vi "Test PJVS.vi"(8 "error in (pass through)":errorcluster, 11 "PJVS setup":T1={"PJVS type"=enum."AC-supraVOLTcontrol", "Status Refnum"=refnum, "Abort Refnum"=refnum, "AC-supraVOLTcontrol"={"IP address:port (0.0.0.0:0000)"="0.0.0.0:0000", "Timeouts"={"TCP Read & Write (ms)"=7000, "Sensors readout"=5000, "PJVS setup"=10000, "Nullmeter readout"=5000, "Multiplexer setup"=3000, "57XX setup"=15000, "Generator setup"=5000, "Synthesizer setup"=3000, "Sampler readout"=10000}, "Simulation mode"=FALSE, "Debug mode"=FALSE}, "NPL bias source"={"Server name"="CZC", "Bias setup file"=path ""}}) -> (0 "error out":errorcluster, 2 "Status":string, 3 "PJVS setup out":T1={"PJVS type"=enum."AC-supraVOLTcontrol", "Status Refnum"=refnum, "Abort Refnum"=refnum, "AC-supraVOLTcontrol"={"IP address:port (0.0.0.0:0000)"="0.0.0.0:0000", "Timeouts"={"TCP Read & Write (ms)"=7000, "Sensors readout"=5000, "PJVS setup"=10000, "Nullmeter readout"=5000, "Multiplexer setup"=3000, "57XX setup"=15000, "Generator setup"=5000, "Synthesizer setup"=3000, "Sampler readout"=10000}, "Simulation mode"=FALSE, "Debug mode"=FALSE}, "NPL bias source"={"Server name"="CZC", "Bias setup file"=path ""}})   [LabVIEW 2020]
doc: "Initialize the PJVS. Calls the initialization routine of the actual driver."
uses:
  Type definitions/PJVS Setup.ctl
  Type definitions/PJVS Type.ctl
  PJVS drivers/acsvcontrol-driver/build/ACSVcontrol-driver_0.2.0.0.llb/Timeouts.ctl
  <vilib>/Utility/error.llb/DialogType.ctl
  PJVS drivers/acsvcontrol-driver/build/ACSVcontrol-driver_0.2.0.0.llb/ACSVcontrol-driver.lvlib
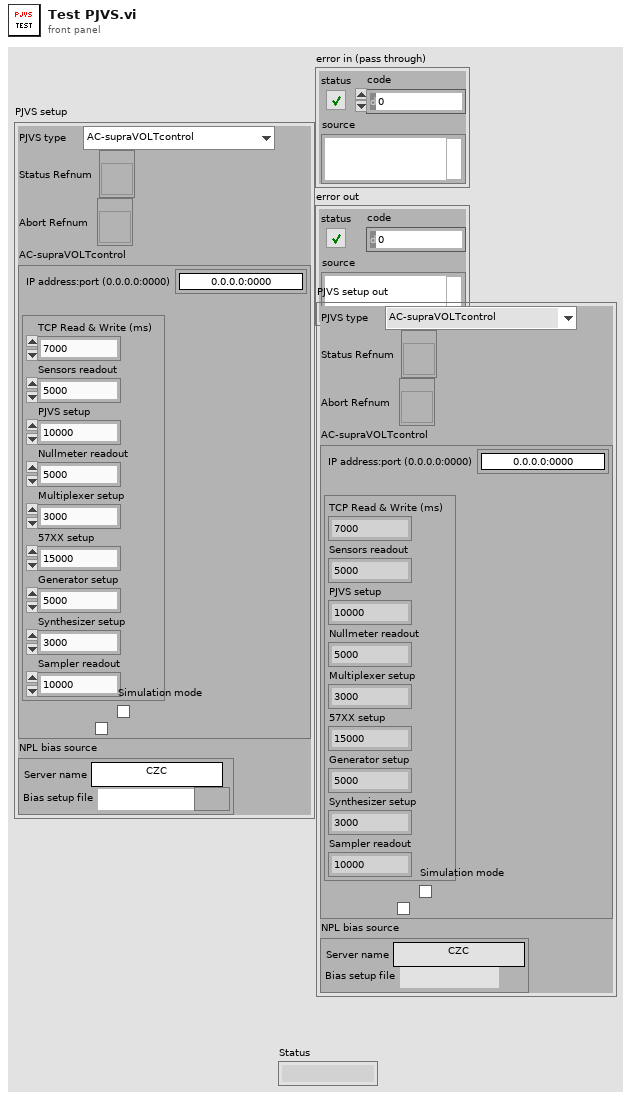
[diagram p1: front panel]
types:
  T1 = typedef "PJVS Setup.ctl" = cluster{"PJVS type":T2, "Status Refnum":refnum<vi>, "Abort Refnum":refnum<vi>, "AC-supraVOLTcontrol":cluster{"IP address:port (0.0.0.0:0000)":string, "Timeouts":T3, "Simulation mode":bool, "Debug mode":bool}, "NPL bias source":cluster{"Server name":string, "Bias setup file":path}}
  T2 = typedef "PJVS Type.ctl" = enum16{"AC-supraVOLTcontrol", "NPL bias source"}
  T3 = typedef "ACSVcontrol-driver.lvlib/Timeouts.ctl" = cluster{"TCP Read & Write (ms)":i32, "Sensors readout":i32, "PJVS setup":i32, "Nullmeter readout":i32, "Multiplexer setup":i32, "57XX setup":i32, "Generator setup":i32, "Synthesizer setup":i32, "Sampler readout":i32}
  T4 = typedef "DialogType.ctl" = u16
  T5 = typedef "ACSVcontrol-driver.lvlib/Sensors Data.ctl" = cluster{"Temperature (°C)":dbl, "Barometric Pressure (mbar)":dbl, "Humidity (%)":dbl, "Temperature Cooler (K)":dbl}
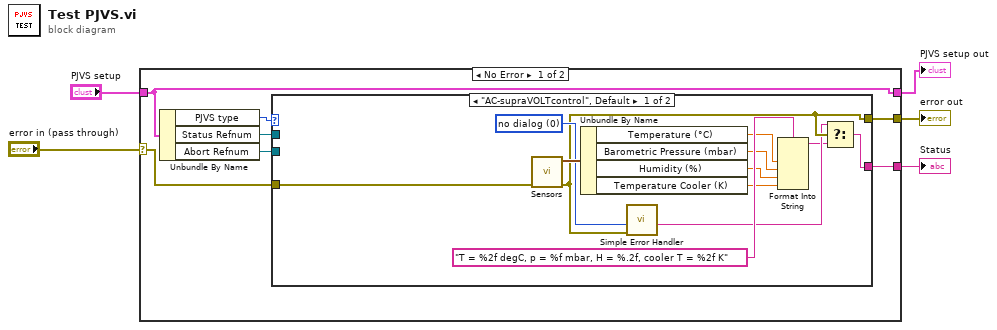
[diagram p0: block diagram]
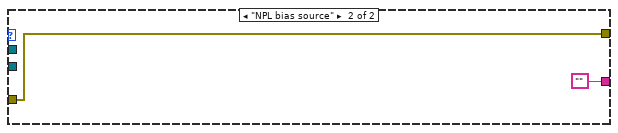
[diagram p2: hidden frame]
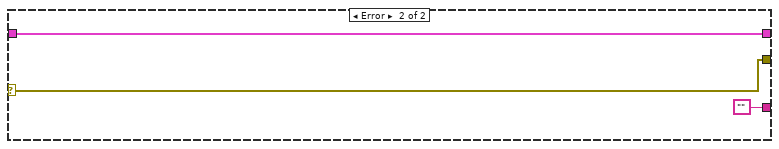
[diagram p3: hidden frame]
diagram:
  n1 = case shown="No Error" "error in (pass through)" {
    selector: "error in (pass through)" -> [w8 w29]
    tunnel: "PJVS setup" -> [w7 w28]
    tunnel: [w9 w29] -> w4
    tunnel: [w7 w28] -> w2
    tunnel: [w6 ""] -> w1
    frame No Error {
      n2 = Unbundle By Name(w7) -> ("PJVS type"=w12:T2, "Status Refnum"=w11:refnum<vi>, "Abort Refnum"=w10:refnum<vi>)
      n3 = case shown="\"AC-supraVOLTcontrol\", Default" w12 {
        tunnel: w11 -> [_ _]
        tunnel: w10 -> [_ _]
        tunnel: w8 -> [w24 w26]
        tunnel: [w16 w26] -> w9
        tunnel: [w13 ""] -> w6
        frame "AC-supraVOLTcontrol", Default {
          w17 = T4 0 items=["no dialog", "OK message", "continue or stop message", "OK message + warnings", "continue/stop + warnings"] ("type of dialog (OK msg:1)")
          n4 = call "Sensors.vi"("error in (no error)"=w24) -> ("error out"=w16:errorcluster, "Sensors Data"=w22:T5)  [unwired: 9 in]
          n5 = Unbundle By Name(w22) -> ("Temperature (°C)"=w21:dbl, "Barometric Pressure (mbar)"=w20:dbl, "Humidity (%)"=w19:dbl, "Temperature Cooler (K)"=w18:dbl)
          n6 = call <vilib>:"Simple Error Handler.vi"("type of dialog (OK msg:1)"=w17, "error in (no error)"=w16) -> ("source out"=w15:string)  [unwired: 3 in, 4 out]
          n7 = Format Into String(format string="T = %2f degC, p = %f mbar, H = %.2f, cooler T = %2f K", w21, w20, w19, w18) -> (resulting string=w14:string)  [unwired: 2 in, 1 out]
          n8 = Select(t=w15, s=w16, f=w14) -> (s? t:f=w13:string)
        }
        frame "NPL bias source" {
        }
      }
    }
    frame Error {
    }
  }
  "error out" <- w4
  "PJVS setup out" <- w2
  "Status" <- w1
